vi "test_Get FPGA Bitfile.vi"(8 "error in (no error)":errorcluster, 11 "TestCase in":refnum<class "FPGA Addon Scripting API Unit Tests.lvclass">) -> (0 "error out":errorcluster, 3 "TestCase out":refnum<class "FPGA Addon Scripting API Unit Tests.lvclass">)   [LabVIEW 2020, in "FPGA Addon Scripting API Unit Tests.lvclass"]
uses:
  FPGA Addon Scripting API Unit Tests.lvclass
  APIs/Scripting API/TypeDefs/Output Scalar Data.ctl
  Addon/Addon Shared/Types/FPGA Addon Data Type.ctl
  <vilib>/addons/_JKI Toolkits/VI Tester/TestCase.llb/TestCase.lvclass
  FPGA Addon Test Class/FPGA Addon Test Class.lvclass
  APIs/Scripting API/Scripting API.lvlib
  Addon/Addon Shared/FPGA Addon Shared.lvlib
  C:/Program Files (x86)/National Instruments/LabVIEW 2020/vi.lib/addons/_JKI Toolkits/VI Tester/TestCase.llb/TestCase.lvclass
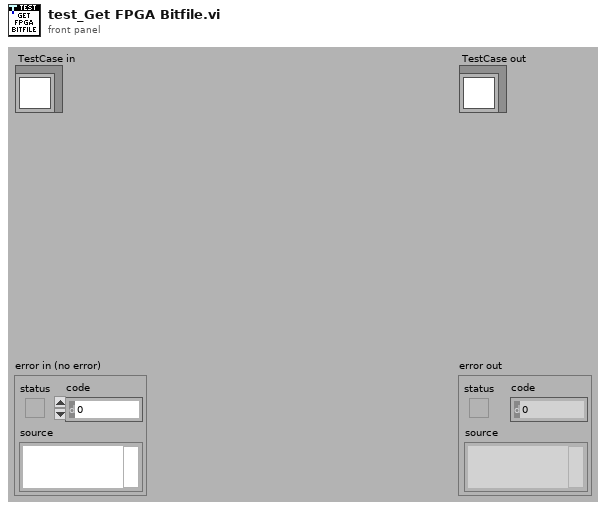
[diagram p1: front panel]
types:
  T1 = typedef "Scripting API.lvlib/Output Scalar Data.ctl" = cluster{"Bitfile Name":string, "SysDef Channel Name":string, "Imported":bool, "Data Type":T2}
  T2 = typedef "FPGA Addon Shared.lvlib/FPGA Addon Data Type.ctl" = enum8{"<Null>", "I8", "I16", "I32", "I64", "U8", "U16", "U32", "U64", "SGL", "Boolean", "Analog PWM In Settings", "Analog PWM In", "Digital PWM In Settings", "Digital PWM In", "Digital PWM Out", "Sine Out", "FXP", "FXP+/-24.5", "FXP+/-16.5", "FXP+/-32.8", "FXP+/-64.32", "FXP+/-16.7", "FXP+/-20.5", "FXP+/-27.5", "FXP+/-32.16", "FXP+16.3", "FXP+18.3", "Digital Static In", "Digital Static Out", "Digital Static In Settings", "Digital WSS Out", "Quad Encoder Settings", "Quad Encoder In", "Group"}
  T3 = typedef "Custom Device API.lvlib/Custom Device Item Ref.ctl" = u64
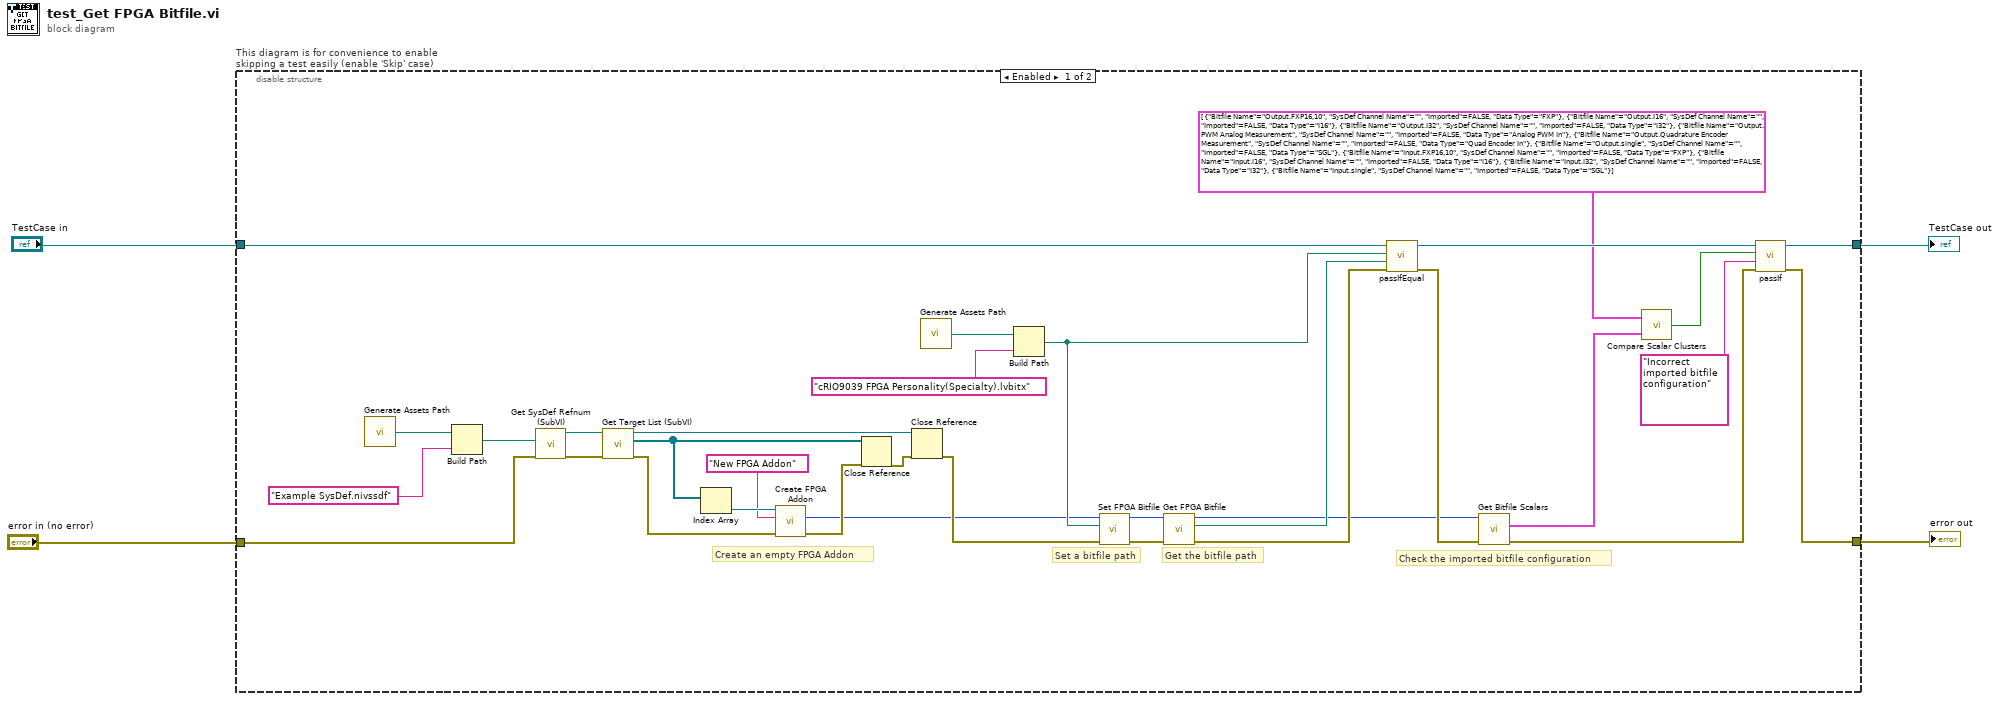
[diagram p0: block diagram]
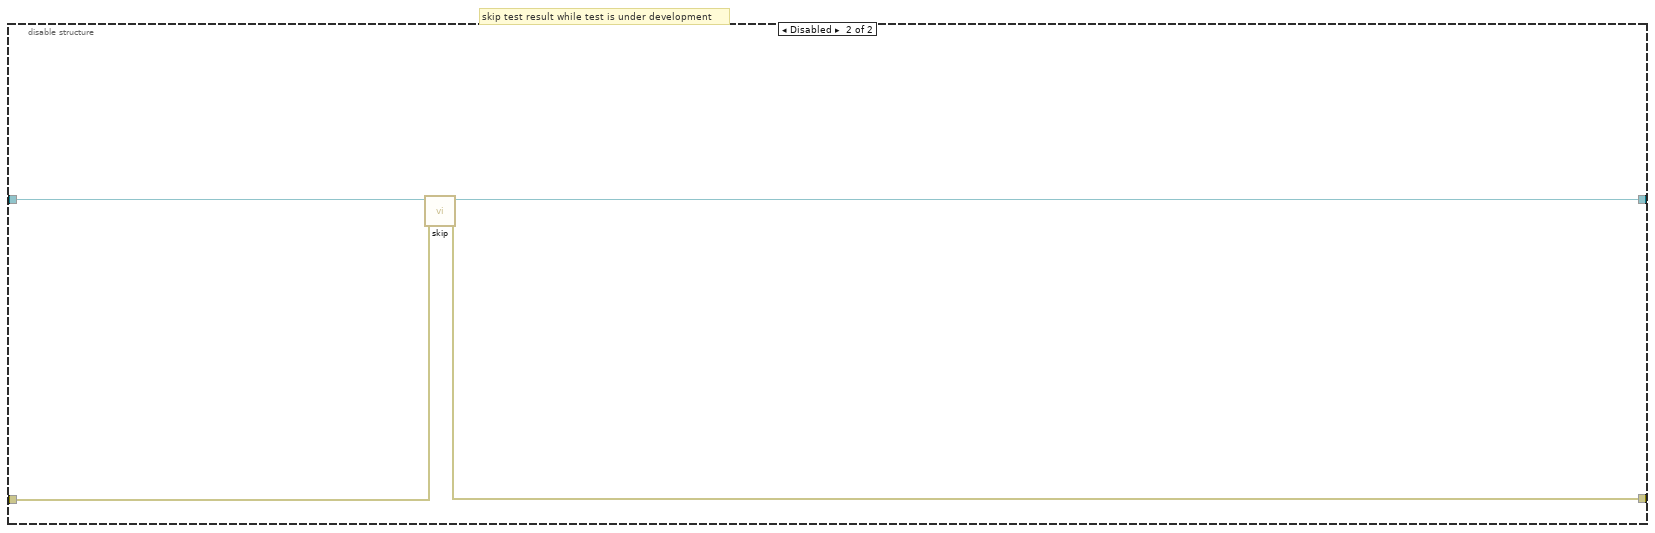
[diagram p2: hidden frame]
diagram:
  n1 = disable-structure "This diagram is for convenience to enable skipping a test easily (enable 'Skip' case)" shown="Enabled" {
    disable-tunnel: "TestCase in" -> [w26 w41]
    disable-tunnel: [w19 w39] -> w1
    disable-tunnel: [w17 w40] -> w3
    disable-tunnel: "error in (no error)" -> [w33 w38]
    frame Enabled {
      # "Get the bitfile path"
      # "Set a bitfile path"
      # "Check the imported bitfile configuration"
      # "Create an empty FPGA Addon"
      n2 = call "Generate Assets Path.vi"() -> ("Assets path"=w37:path)
      n3 = Build Path(base path=w37, name or relative path="Example SysDef.nivssdf") -> (appended path=w35:path)
      n4 = call "Get SysDef Refnum (SubVI).vi"("error in (no error)"=w33, "System Definition path"=w35) -> ("error out"=w32:errorcluster, "SysDef Refnum out"=w34:refnum<k24>)  [unwired: 8 in]
      n5 = call "Get Target List (SubVI).vi"("error in (no error)"=w32, "SysDef Refnum in"=w34) -> ("error out"=w9:errorcluster, "Target List Refnums"=w31:refnum<k24>[], "SysDef Refnum out"=w30:refnum<k24>)  [unwired: 7 in]
      n6 = Index Array(array=w31) -> (element=w10:refnum<k24>)  [unwired: 1 in]
      n7 = call "Create FPGA Addon.vi"("error in"=w9, "FPGA addon name"="New FPGA Addon", "target in"=w10) -> ("error out"=w7:errorcluster, "FPGA addon refnum"=w6:T3)  [unwired: 6 in, 1 out]
      n8 = Close Reference(reference=w31, error in (no error)=w7) -> (error out=w29:errorcluster)
      n9 = Close Reference(reference=w30, error in (no error)=w29) -> (error out=w14:errorcluster)
      n10 = call "Generate Assets Path.vi"() -> ("Assets path"=w28:path)
      n11 = Build Path(base path=w28, name or relative path="cRIO9039 FPGA Personality(Specialty).lvbitx") -> (appended path=w11:path)
      n12 = call "Set FPGA Bitfile.vi"("error in"=w14, "FPGA bitfile path"=w11, "FPGA addon refnum in"=w6) -> ("error out"=w13:errorcluster, "FPGA addon refnum out"=w12:T3)  [unwired: 7 in]
      n13 = call "Get FPGA Bitfile.vi"("error in"=w13, "FPGA addon refnum in"=w12) -> ("error out"=w24:errorcluster, "FPGA bitfile path"=w25:path, "FPGA addon refnum out"=w22:T3)  [unwired: 7 in]
      n14 = call-dynamic "passIfEqual.vi"("error in (no error)"=w24, "y"=w25, "x"=w11, "TestCase in"=w26) -> ("error out"=w23:errorcluster, "TestCase out"=w20:refnum<class "FPGA Addon Scripting API Unit Tests.lvclass">)  [unwired: 6 in]
      n15 = call "Get Bitfile Scalars.vi"("error in"=w23, "FPGA addon refnum in"=w22) -> ("error out"=w18:errorcluster, "bitfile scalars out"=w21:T1[])  [unwired: 7 in, 1 out]
      n16 = call "Compare Scalar Clusters.vi"("Target bitfile scalars in"=w21, "Reference bitfile scalars in"=T1[] [{"Bitfile Name"="Output.FXP16,10", "SysDef Channel Name"="", "Imported"=FALSE, "Data Type"=enum."FXP"}, {"Bitfile Name"="Output.I16", "SysDef Channel Name"="", "Imported"=FALSE, "Data Type"=enum."I16"}, {"Bitfile Name"="Output.I32", "SysDef Channel Name"="", "Imported"=FALSE, "Data Type"=enum."I32"}, {"Bitfile Name"="Output.PWM Analog Measurement", "SysDef Channel Name"="", "Imported"=FALSE, "Data Type"=enum."Analog PWM In"}, {"Bitfile Name"="Output.Quadrature Encoder Measurement", "SysDef Channel Name"="", "Imported"=FALSE, "Data Type"=enum."Quad Encoder In"}, {"Bitfile Name"="Output.single", "SysDef Channel Name"="", "Imported"=FALSE, "Data Type"=enum."SGL"}, {"Bitfile Name"="Input.FXP16,10", "SysDef Channel Name"="", "Imported"=FALSE, "Data Type"=enum."FXP"}, {"Bitfile Name"="Input.I16", "SysDef Channel Name"="", "Imported"=FALSE, "Data Type"=enum."I16"}, {"Bitfile Name"="Input.I32", "SysDef Channel Name"="", "Imported"=FALSE, "Data Type"=enum."I32"}, {"Bitfile Name"="Input.single", "SysDef Channel Name"="", "Imported"=FALSE, "Data Type"=enum."SGL"}] ("bitfile scalars out")) -> ("Equal ?"=w16:bool)
      n17 = call-dynamic "passIf.vi"("error in (no error)"=w18, "message (\"\")"="Incorrect imported bitfile configuration" ("message (\"\")"), "pass"=w16, "TestCase in"=w20) -> ("error out"=w17:errorcluster, "TestCase out"=w19:refnum<class "FPGA Addon Scripting API Unit Tests.lvclass">)  [unwired: 6 in]
    }
    frame Disabled {
      # "skip test result while test is under development"
      n18 = call <vilib>:"skip.vi"("error in (no error)"=w38, "TestCase in"=w41) -> ("error out"=w40:errorcluster, "TestCase out"=w39:refnum<class "FPGA Addon Scripting API Unit Tests.lvclass">)  [unwired: 8 in]
    }
  }
  "error out" <- w3
  "TestCase out" <- w1
